vi "Load Device Class.vi"(11 "Abstract Spectrometer in":refnum<class "Abstract Spectrometer.lvclass">) -> (0 "error out":errorcluster, 3 "Abstract Spectrometer out":refnum<class "Abstract Spectrometer.lvclass">)   [LabVIEW 2019, in "Spectrometer.lvlib"]
uses:
  Spectrometer.lvlib
  Spectrometer-LVClass/Abstract Spectrometer_class/Abstract Spectrometer.lvclass
  Spectrometer-LVClass/Simulated_class/Simulated.lvclass
  G:/LabVIEW/Spectrometer-LVClass/Abstract Spectrometer_class/Abstract Spectrometer.lvclass
  Spectrometer-LVClass/SpectraPro_class/SpectraPro.lvclass
  <vilib>/Utility/config.llb/Read Key (I32).vi
  <vilib>/Utility/config.llb/NI_LVConfig.lvlib
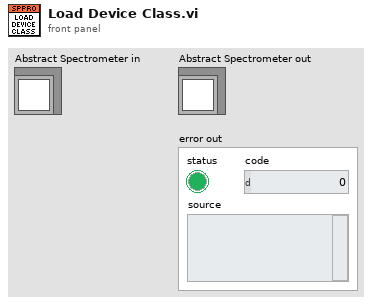
[diagram p1: front panel]
types:
  T1 = typedef "NI_LVConfig.lvlib/Config Data RefNum.ctl" = refnum<k1>
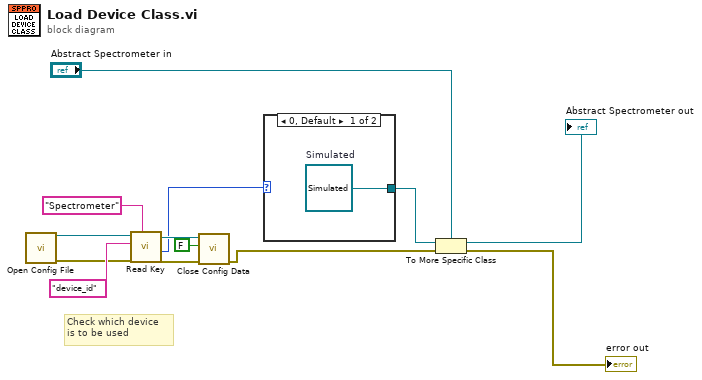
[diagram p0: block diagram]
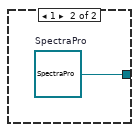
[diagram p2: hidden frame]
diagram:
  # "Check which device\nis to be used"
  n1 = call "Open Config File.vi"() -> ("error out"=w5:errorcluster, "Refnum out"=w6:T1)  [unwired: 10 in]
  n2 = call-poly <vilib>:"Read Key.vi"("section"="Spectrometer", "error in (no error)"=w5, "key"="device_id", "refnum"=w6) -> ("error out"=w12:errorcluster, "value"=w9:i32, "refnum out"=w11:T1)  [unwired: 4 in, 1 out]
  n3 = call <vilib>:"Close Config Data.vi"("error in (no error)"=w12, "write file if changed (T)"=FALSE, "refnum"=w11) -> ("error out"=w13:errorcluster)  [unwired: 7 in, 1 out]
  n4 = case shown="0, Default" w9 {
    tunnel: [w14 w15] -> w4
    frame 0, Default {
      w14 = refnum<class "Simulated.lvclass"> refnum  # Simulated
    }
    frame 1 {
      w15 = refnum<class "SpectraPro.lvclass"> refnum  # SpectraPro
    }
  }
  n5 = To More Specific Class(target class="Abstract Spectrometer in", reference=w4, error in=w13) -> (specific class reference=→"Abstract Spectrometer out":refnum<class "Abstract Spectrometer.lvclass">, error out=→"error out":errorcluster)
